vi "Clear.vi"(8 "error in (no error)":errorcluster, 11 "Execution UI In":refnum<class "Execution UI V2.lvclass">) -> (0 "error out":errorcluster, 3 "Execution UI Out":refnum<class "Execution UI V2.lvclass">)   [LabVIEW 2020, in "Execution UI V2.lvclass"]
uses:
  Execution UI V2.lvclass
  Execution UI V2.lvclass/Execution UI V2.ctl
  Application Framework/Process Classes/Process/Process.lvclass
  Result Model/Result Model.lvclass
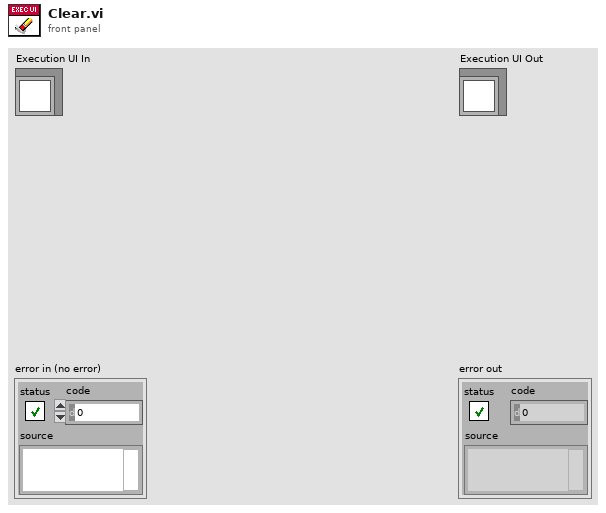
[diagram p1: front panel]
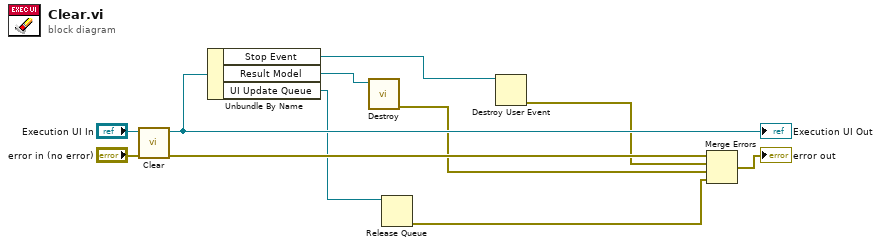
[diagram p0: block diagram]
diagram:
  n1 = call-parent "Clear.vi"("error in (no error)"="error in (no error)", "Process In"="Execution UI In") -> ("error out"=w11:errorcluster, "Process Out"=w8:refnum<class "Execution UI V2.lvclass">)  [unwired: 8 in]
  "Execution UI Out" <- w8
  n2 = Unbundle By Name(w8) -> ("Stop Event"=w6:refnum<user-event>, "Result Model"=w4:refnum<class "Result Model.lvclass">, "UI Update Queue"=w2:refnum<queue>)
  n3 = call "Destroy.vi"("Result Model in"=w4) -> ("error out"=w3:errorcluster)  [unwired: 10 in]
  n4 = Release Queue(queue=w2) -> (error out=w1:errorcluster)  [unwired: 2 in, 2 out]
  n5 = Destroy User Event(user event=w6) -> (error out=w5:errorcluster)  [unwired: 1 in]
  n6 = Merge Errors(w11, w5, w3, w1) -> (→"error out":errorcluster)
